vi "DoEat.vi"(8 "error in (no error)":errorcluster, 10 "SnakeGame in":refnum<class "SnakeGame.lvclass">, 11 "Snake in":refnum<class "Snake.lvclass">) -> (0 "error out":errorcluster, 2 "SnakeGame out":refnum<class "SnakeGame.lvclass">, 3 "Snake out":refnum<class "Snake.lvclass">)   [LabVIEW 2019, in "RT_Game.lvlib" / "Snake.lvclass"]
uses:
  Snake.lvclass
  SnakeGame/SnakeGame.lvclass
  C:/Users/FreshBob/Dropbox/VIs/myRIO_GameConsole/RT/RT_Game/Game/Game.lvclass
  Snake.lvclass/Snake.ctl
  SnakeGame/SnakeGame.lvclass/SnakeGame.ctl
  GameObject/GameObject.lvclass/GameObject.ctl
  PongSwitch/SnakeSwitch.lvclass/SnakeSwitch.ctl
  GameObject/Read position.vi
  PongSwitch/Write Tilecode.vi
  GameObject/Write IsActive.vi
  GameObject/Read name.vi
  GameObject/Read IsActive.vi
  PongSwitch/Read Toggled.vi
  SnakeGame/Read Switches.vi
  SnakeGame/Read Snakes.vi
  Read Position (Tiles).vi
  SnakeGame/Write Switches.vi
  PongSwitch/SnakeSwitch.lvclass
  C:/Users/FreshBob/Dropbox/VIs/myRIO_GameConsole/RT/RT_Game/GameObject/GameObject.lvclass
  Game/Game.lvclass
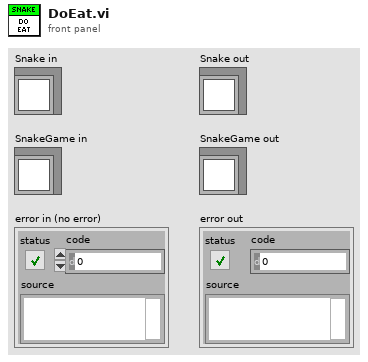
[diagram p1: front panel]
types:
  T1 = typedef "RT_Game.lvlib/Game.lvclass/Coordinate.ctl" = cluster{"x":dbl, "y":dbl}
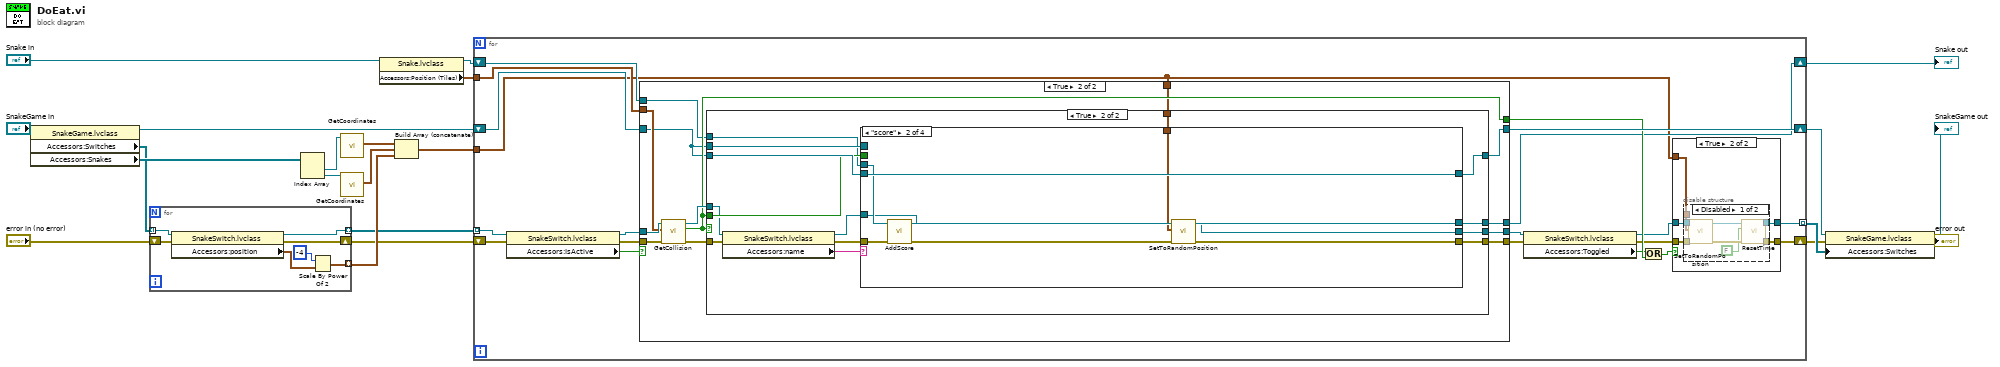
[diagram p0: block diagram]
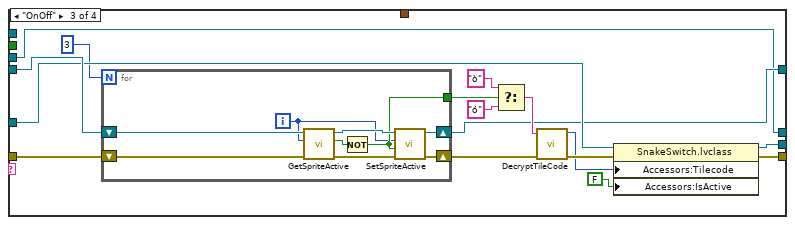
[diagram p7: hidden frame]
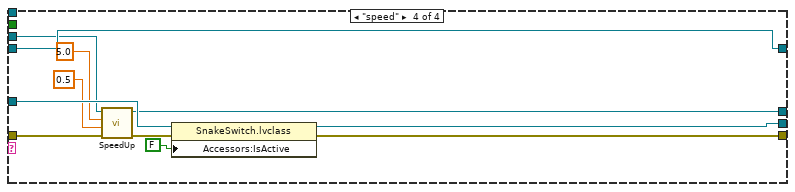
[diagram p8: hidden frame]
diagram:
  n1 = property class="SnakeGame.lvclass"(reference="SnakeGame in") -> (reference out=w8:refnum<class "SnakeGame.lvclass">, "Accessors:Switches"=w10:refnum<class "SnakeSwitch.lvclass">[], "Accessors:Snakes"=w11:refnum<class "Snake.lvclass">[])  [unwired: 1 in, 1 out]
  n2 = for {
    tunnel: [w27] -> w5 mode=indexing
    tunnel: w10 -> [w26] mode=indexing
    shift-right: [w28] -> w6
    shift-left: "error in (no error)" -> [w29]
    tunnel: [w24] -> w7 mode=indexing
    n3 = property class="SnakeSwitch.lvclass"(reference=w26, error in=w29) -> (reference out=w27:refnum<class "SnakeSwitch.lvclass">, error out=w28:errorcluster, "Accessors:position"=w25:T1)
    n4 = Scale By Power Of 2(n=i16 -4, x=w25) -> (x*2^n=w24:T1)
  }
  n5 = Index Array(array=w11) -> (element #1=w18:refnum<class "Snake.lvclass">, element #2=w1:refnum<class "Snake.lvclass">)  [unwired: 2 in]
  n6 = call "GetCoordinates.vi"("Snake in"=w18) -> ("Coordinates"=w3:T1[])  [unwired: 8 in, 2 out]
  n7 = call "GetCoordinates.vi"("Snake in"=w1) -> ("Coordinates"=w2:T1[])  [unwired: 8 in, 2 out]
  n8 = property class="Snake.lvclass"(reference="Snake in") -> (reference out=w21:refnum<class "Snake.lvclass">, "Accessors:Position (Tiles)"=w20:T1)  [unwired: 1 in, 1 out]
  n9 = Build Array (concatenate)(w3, w2, w7) -> (w4:T1[])
  n10 = for {
    shift-right: [w31] -> w13
    shift-left: w6 -> [w39]
    shift-right: [w48] -> w14
    shift-left: w8 -> [w47]
    tunnel: w5 -> [w40] mode=indexing
    tunnel: w20 -> [w49]
    tunnel: w4 -> [w30]
    tunnel: [w41] -> w16 mode=indexing
    shift-right: [w37] -> w22
    shift-left: w21 -> [w38]
    n11 = property class="SnakeSwitch.lvclass"(reference=w40, error in=w39) -> (reference out=w45:refnum<class "SnakeSwitch.lvclass">, error out=w46:errorcluster, "Accessors:IsActive"=w44:bool)
    n12 = case shown="True" w44 {
      tunnel: w46 -> [w69 w83]
      tunnel: w45 -> [w70 w82]
      tunnel: w49 -> [_ w79]
      tunnel: [w69 w78] -> w43
      tunnel: [w70 w77] -> w35
      tunnel: [w68 w76] -> w48
      tunnel: w47 -> [w68 w74]
      tunnel: [_ w75] -> w42
      tunnel: w38 -> [w67 w73]
      tunnel: [w67 w72] -> w37
      tunnel: w30 -> [_ w71]
      frame False {
      }
      frame True {
        n13 = call "GetCollision"("error in (no error)"=w83, "TilePosition"=w79, "PongSwitch in"=w82) -> ("error out"=w80:errorcluster, "Collided?"=w75:bool, "PongSwitch out"=w81:refnum<class "SnakeSwitch.lvclass">)  [unwired: 6 in]
        n14 = case shown="True" w75 {
          tunnel: w80 -> [w86 w91]
          tunnel: [w86 w101] -> w78
          tunnel: w81 -> [w87 w92]
          tunnel: [w87 w93] -> w77
          tunnel: [w85 w99] -> w76
          tunnel: w74 -> [w85 w100]
          tunnel: w75 -> [_ w96]
          tunnel: w74 -> [_ w95]
          tunnel: w73 -> [w84 w90]
          tunnel: [w84 w89] -> w72
          tunnel: w71 -> [_ w88]
          frame False {
          }
          frame True {
            n15 = property class="SnakeSwitch.lvclass"(reference=w92, error in=w91) -> (reference out=w94:refnum<class "SnakeSwitch.lvclass">, error out=w98:errorcluster, "Accessors:name"=w97:string)
            n16 = case shown="\"score\"" w97 {
              tunnel: w98 -> [w104 w110 w130 w143]
              tunnel: [w104 w109 w127 w150] -> w101
              tunnel: w100 -> [w105 w114 w128 w146]
              tunnel: [w105 w114 w118 w146] -> w99
              tunnel: w96 -> [_ _ _ _]
              tunnel: w95 -> [_ _ _ _]
              tunnel: w94 -> [w103 w108 w126 w148]
              tunnel: [w103 w107 w117 w149] -> w93
              tunnel: w90 -> [w102 w113 w115 w140]
              tunnel: [w102 w112 w115 w141] -> w89
              tunnel: w88 -> [_ w106 _ _]
              frame Default {
              }
              frame "score" {
                n17 = call "AddScore.vi"("error in (no error)"=w110, "Snake in"=w113) -> ("error out"=w111:errorcluster, "Snake out"=w112:refnum<class "Snake.lvclass">)  [unwired: 8 in]
                n18 = call "SetToRandomPosition.vi"("error in (no error)"=w111, "BlockedSpots"=w106, "SnakeSwitch in"=w108) -> ("error out"=w109:errorcluster, "SnakeSwitch out"=w107:refnum<class "SnakeSwitch.lvclass">)  [unwired: 7 in]
              }
              frame "OnOff" {
                n19 = for {
                  N: 3 -> [_]
                  tunnel: [w132] -> w121
                  shift-right: [w138] -> w129
                  shift-left: w130 -> [w139]
                  shift-right: [w137] -> w118
                  shift-left: w128 -> [w135]
                  i -> [w131]
                  n20 = call "GetSpriteActive.vi"("error in (no error)"=w139, "Index"=w131, "Game in"=w135) -> ("error out"=w136:errorcluster, "Active?"=w133:bool, "Game out"=w134:refnum<class "SnakeGame.lvclass">)  [unwired: 6 in]
                  n21 = Not(x=w133) -> (.not. x?=w132:bool)
                  n22 = call "SetSpriteActive.vi"("error in (no error)"=w136, "Active"=w132, "index"=w131, "Game in"=w134) -> ("error out"=w138:errorcluster, "Game out"=w137:refnum<class "SnakeGame.lvclass">)  [unwired: 6 in]
                }
                n23 = Select(t="ò" ("f"), s=w121, f="ó" ("TileCode")) -> (s? t:f=w124:string)
                n24 = call "DecryptTileCode.vi"("error in (no error)"=w129, "TileCode"=w124) -> ("error out"=w125:errorcluster, "TileCode"=w120:u16)  [unwired: 6 in, 2 out]
                n25 = property class="SnakeSwitch.lvclass"(reference=w126, error in=w125, "Accessors:Tilecode"=w120, "Accessors:IsActive"=FALSE ("IsActive")) -> (reference out=w117:refnum<class "SnakeSwitch.lvclass">, error out=w127:errorcluster)
              }
              frame "speed" {
                n26 = call "SpeedUp.vi"("error in (no error)"=w143, "speed multiplier"=0.5, "Duration"=5.0, "Snake in"=w140) -> ("error out"=w142:errorcluster, "Snake out"=w141:refnum<class "Snake.lvclass">)  [unwired: 6 in]
                n27 = property class="SnakeSwitch.lvclass"(reference=w148, error in=w142, "Accessors:IsActive"=FALSE ("IsActive")) -> (reference out=w149:refnum<class "SnakeSwitch.lvclass">, error out=w150:errorcluster)
              }
            }
          }
        }
      }
    }
    n28 = property class="SnakeSwitch.lvclass"(reference=w35, error in=w43) -> (reference out=w34:refnum<class "SnakeSwitch.lvclass">, error out=w36:errorcluster, "Accessors:Toggled"=w32:bool)
    n29 = Or(x=w32, y=w42) -> (x .or. y?=w33:bool)
    n30 = case shown="True" w33 {
      tunnel: [w50 w53] -> w31
      tunnel: [w51 w52] -> w41
      tunnel: w30 -> [_ w56]
      tunnel: w36 -> [w50 w55]
      tunnel: w34 -> [w51 w54]
      frame False {
      }
      frame True {
        n31 = disable-structure shown="Disabled" {
          disable-tunnel: w56 -> [w63 _]
          disable-tunnel: w55 -> [w62 w65]
          disable-tunnel: w54 -> [w61 w66]
          disable-tunnel: [w60 w65] -> w53
          disable-tunnel: [w58 w66] -> w52
          frame Disabled {
            n32 = call "SetToRandomPosition.vi"("error in (no error)"=w62, "BlockedSpots"=w63, "SnakeSwitch in"=w61) -> ("error out"=w64:errorcluster, "SnakeSwitch out"=w59:refnum<class "SnakeSwitch.lvclass">)  [unwired: 7 in]
            n33 = call "ResetTime.vi"("error in (no error)"=w64, "enabled"=FALSE, "SnakeSwitch in"=w59) -> ("error out"=w60:errorcluster, "SnakeSwitch out"=w58:refnum<class "SnakeSwitch.lvclass">)  [unwired: 7 in]
          }
          frame Enabled {
          }
        }
      }
    }
  }
  "Snake out" <- w22
  n34 = property class="SnakeGame.lvclass"(reference=w14, error in=w13, "Accessors:Switches"=w16) -> (reference out=→"SnakeGame out":refnum<class "SnakeGame.lvclass">, error out=→"error out":errorcluster)
